vi "SR_J-Check A button.vi"(8 "error in (no error)":errorcluster, 10 "RDS Msg Q in":refnum<user-event>, 11 "Joystick":T1) -> (0 "error out":errorcluster, 2 "RDS Msg Q out":refnum<user-event>, 3 "Joystick 2":T1)   [LabVIEW 2015, in "Shore Library.lvlib"]
uses:
  Shore Library.lvlib
  SR-J-State.ctl
  Libraries/RDS Framework/RDS Message Class/RDS Message.lvclass
  Libraries/RDS Child Messages/Controller Message/Controller Message Type.ctl
  Actors/RDS Controller Actor/RDS Controller Actor/Controller.ctl
  Libraries/RDS Child Messages/Controller Message/Controller Message.lvclass
  Actors/RDS Controller Actor/RDS Controller Actor/RDS Controller Actor.lvlib
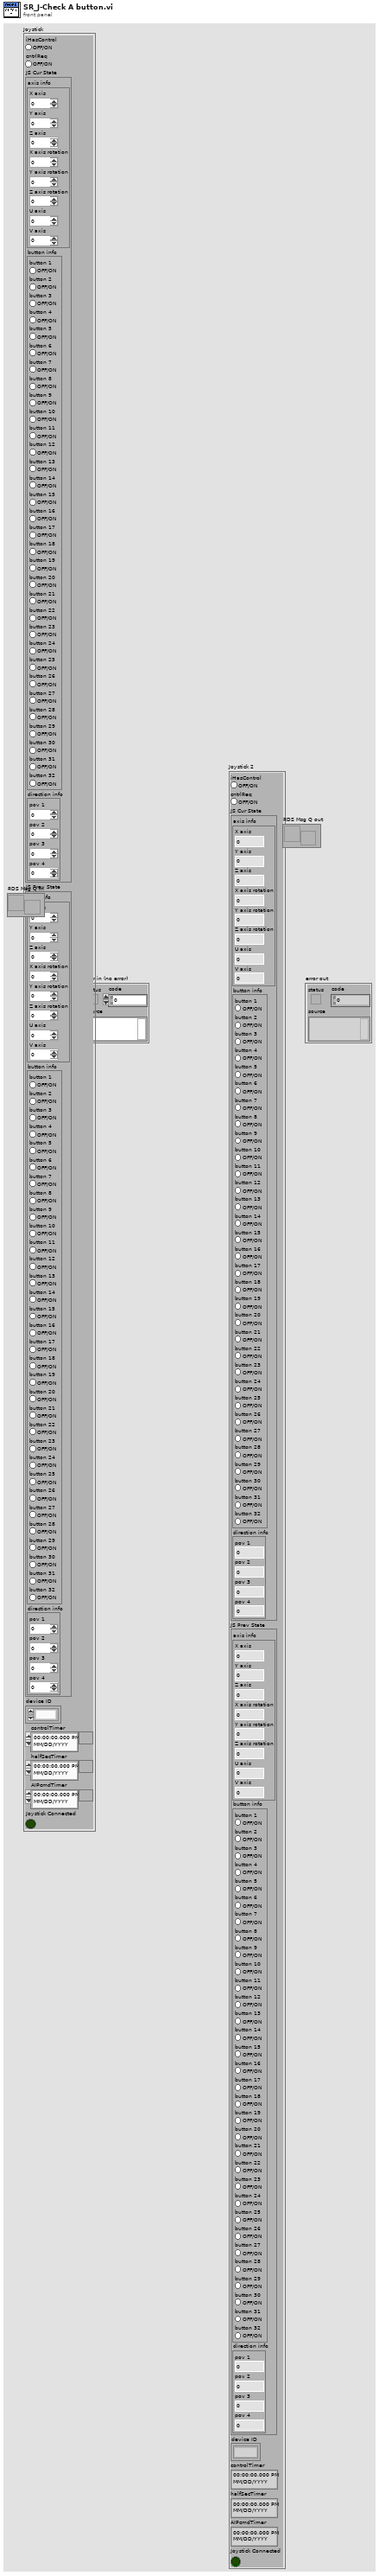
[diagram p1: front panel]
types:
  T1 = typedef "Shore Library.lvlib/SR-J-State.ctl" = cluster{"iHasControl":bool, "cntrlReq":bool, "JS Cur State":cluster{"axis info":cluster{"X axis":i32, "Y axis":i32, "Z axis":i32, "X axis rotation":i32, "Y axis rotation":i32, "Z axis rotation":i32, "U axis":i32, "V axis":i32}, "button info":cluster{"button 1":bool, "button 2":bool, "button 3":bool, "button 4":bool, "button 5":bool, "button 6":bool, "button 7":bool, "button 8":bool, "button 9":bool, "button 10":bool, "button 11":bool, "button 12":bool, "button 13":bool, "button 14":bool, "button 15":bool, "button 16":bool, "button 17":bool, "button 18":bool, "button 19":bool, "button 20":bool, "button 21":bool, "button 22":bool, "button 23":bool, "button 24":bool, "button 25":bool, "button 26":bool, "button 27":bool, "button 28":bool, "button 29":bool, "button 30":bool, "button 31":bool, "button 32":bool}, "direction info":cluster{"pov 1":i32, "pov 2":i32, "pov 3":i32, "pov 4":i32}}, "JS Prev State":cluster{"axis info":cluster{"X axis":i32, "Y axis":i32, "Z axis":i32, "X axis rotation":i32, "Y axis rotation":i32, "Z axis rotation":i32, "U axis":i32, "V axis":i32}, "button info":cluster{"button 1":bool, "button 2":bool, "button 3":bool, "button 4":bool, "button 5":bool, "button 6":bool, "button 7":bool, "button 8":bool, "button 9":bool, "button 10":bool, "button 11":bool, "button 12":bool, "button 13":bool, "button 14":bool, "button 15":bool, "button 16":bool, "button 17":bool, "button 18":bool, "button 19":bool, "button 20":bool, "button 21":bool, "button 22":bool, "button 23":bool, "button 24":bool, "button 25":bool, "button 26":bool, "button 27":bool, "button 28":bool, "button 29":bool, "button 30":bool, "button 31":bool, "button 32":bool}, "direction info":cluster{"pov 1":i32, "pov 2":i32, "pov 3":i32, "pov 4":i32}}, "device ID":refnum<k1>, "controlTimer":timestamp, "halfSecTimer":timestamp, "AIPcmdTimer":timestamp, "Joystick Connected":bool}
  T2 = typedef "RDS Controller Actor.lvlib/Controller.ctl" = enum16{"Idle", "Local Remote Control", "Shore Remote Control", "Mission Control"}
  T3 = typedef "RDS Child Messages.lvlib/Controller Message.lvclass/Controller Message Type.ctl" = enum16{"Control Relinquish Request", "Control Relinquish Command", "Control Request", "Control Granted"}
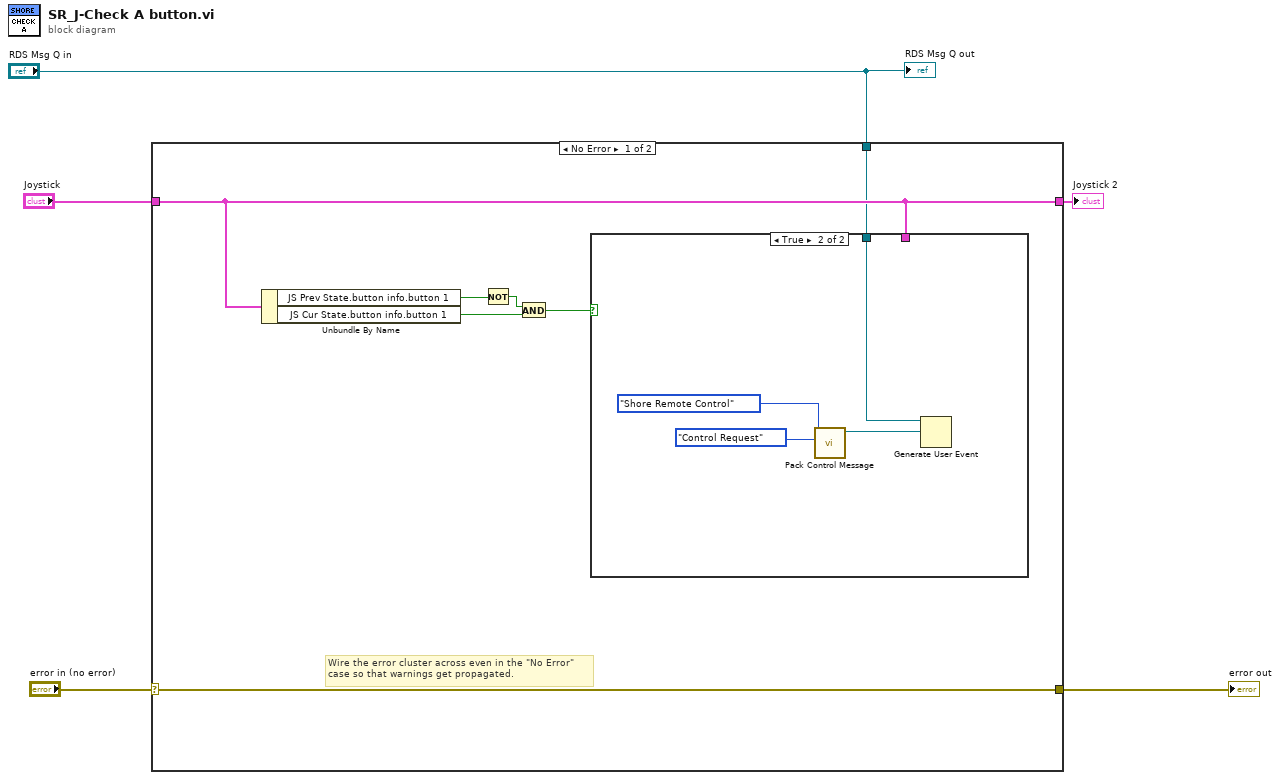
[diagram p0: block diagram]
diagram:
  n1 = case shown="No Error" "error in (no error)" {
    selector: "error in (no error)" -> [w12 w18]
    tunnel: [w12 w18] -> w4
    tunnel: [w7 w17] -> w2
    tunnel: "Joystick" -> [w7 w17]
    tunnel: "RDS Msg Q in" -> [w6 _]
    frame No Error {
      # "Wire the error cluster across even in the \"No Error\"\ncase so that warnings get propagated."
      n2 = Unbundle By Name(w7) -> ("JS Prev State.button info.button 1"=w11:bool, "JS Cur State.button info.button 1"=w9:bool)
      n3 = Not(x=w11) -> (.not. x?=w10:bool)
      n4 = And(x=w10, y=w9) -> (x .and. y?=w8:bool)
      n5 = case shown="True" w8 {
        tunnel: w7 -> [_ _]
        tunnel: w6 -> [_ w15]
        frame False {
        }
        frame True {
          n6 = call "Pack Control Message.vi"("Controller Message Type"=Controller_Message_Type."Control Request", "Controller"=Controller."Shore Remote Control") -> ("Controller Message out"=w14:refnum<class "Controller Message.lvclass">)  [unwired: 9 in]
          n7 = Generate User Event(user event=w15, event data cluster=w14) -> ()  [unwired: 2 in, 2 out]
        }
      }
    }
    frame Error {
    }
  }
  "error out" <- w4
  "Joystick 2" <- w2
  "RDS Msg Q out" <- "RDS Msg Q in"
